vi "Read I16 analogue Data.vi"(6 "Block Header":string, 7 "Channel info":T1[](array[typedef]), 8 "Time Trace In":T2[](array[typedef]), 9 "Analogue Index":i32[](array[numeric]), 10 "pos offset (bytes:0)":i32, 11 "refnum":refnum<file>) -> (0 "Time Trace out":T2[](array[typedef]), 1 "EOF?":bool, 2 "mark after read (bytes)":i32)   [LabVIEW 2021]
uses:
  Controls/Time_Trace_Cluster.ctl
  Controls/Read I16 data cluster.ctl
  Globals/Meas_global.vi
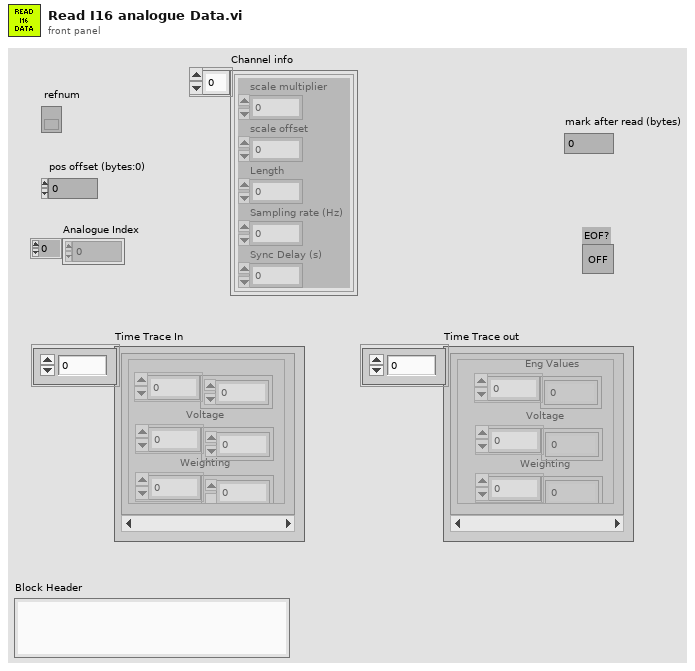
[diagram p1: front panel]
types:
  T1 = typedef "Read I16 data cluster.ctl" = cluster{"scale multiplier":dbl, "scale offset":dbl, "Length":i32, "Sampling rate (Hz)":dbl, "Sync Delay (s)":dbl}
  T2 = typedef "Time_Trace_Cluster.ctl" = cluster{"Weighting":dbl[], "Voltage":dbl[], "Eng Values":dbl[]}
  T3 = typedef "Analysis_info_cluster.ctl" = cluster{"Colour":u32, "Inst type":T4, "Inst name":string, "Symbol":string, "Code name":string, "Extra Info":string, "Inst Array":T5, "Extra Titles":string[], "Extra Values":string[], "U":dbl, "u^2":dbl, "u^3":dbl, "u^4":dbl, "Skew_u":dbl, "Kurt_u":dbl, "Sd Error in Mean":dbl, "% u'/U":dbl, "X":dbl, "Y":dbl, "Z":dbl, "Timescale integral Estimate":dbl, "Sd Error in Variance":dbl, "Calib File":path, "Calib Constants":dbl[], "Output Position":bool, "Stats":enum16{"None", "Basic", "Full"}, "Av Sampling Rate":dbl, "Av No of Samples":dbl, "Total Meas Time (s)":dbl, "ADAM Ch Name":string, "Max value":dbl, "Min value":dbl, "Req Sample Rate Hz":dbl, "Sync Delay Time (s)":dbl, "Ch No":i16, "Device":string, "Use Latest Calib":bool, "Port":string, "Metadata Ch Names":string[], "Metadata Ch Values":string[], "Label":string}
  T4 = typedef "Inst_type.ctl" = enum16{"Raw voltage", "Raw with zero offsetting", "Propeller anemometer", "Pressure Transducer", "Pitot-static tube", "Hot wire", "Cross wire 1", "Cross wire 2", "Generic Linear", "Generic Polynomial", "Generic BackPoly", "Fast FID", "Thermocouple", "Cold wire", "Pulsed Wire", "LDA Vel", "LDA Tran time", "LDA Arr time", "Microphone"}
  T5 = typedef "Instrument_Array.ctl" = enum16{"PWA", "LDA", "Analogue"}
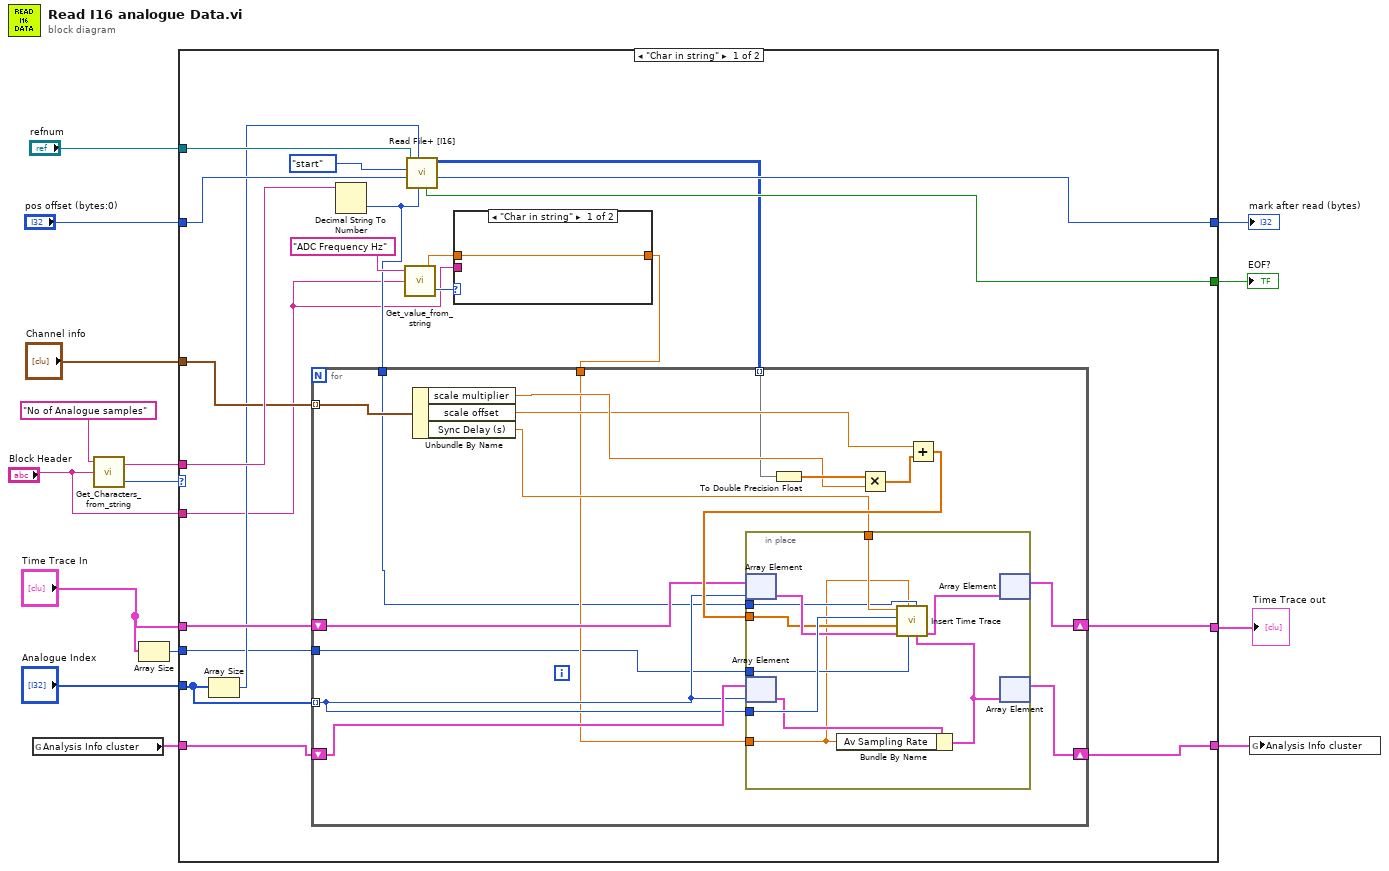
[diagram p0: block diagram]
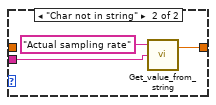
[diagram p2: hidden frame]
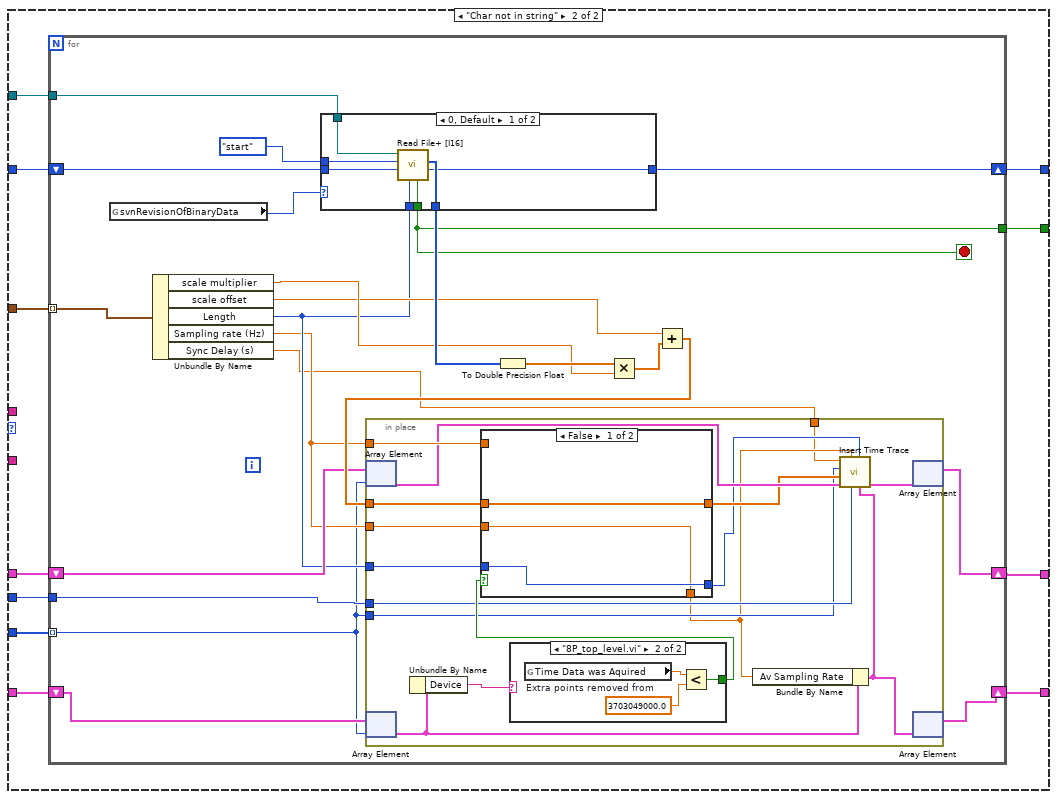
[diagram p3: hidden frame]
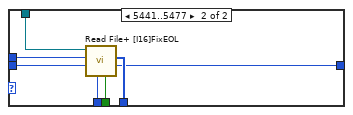
[diagram p4: hidden frame]
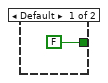
[diagram p5: hidden frame]
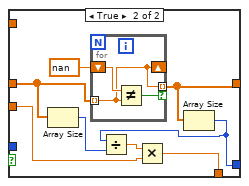
[diagram p6: hidden frame]
diagram:
  n1 = global read "Meas_global.vi" "Analysis Info cluster"() -> (w2:T3[])
  n2 = call "Get_Characters_from_string.vi"("Input string"="Block Header", "Variable name"="No of Analogue samples") -> ("Status"=w8:enum16{"Char in string", "Char not in string"}, "Value"=w7:string)  [unwired: 1 in]
  n3 = Array Size(array="Time Trace In") -> (size(s)=w3:i32)
  n4 = case shown="\"Char in string\"" w8 {
    tunnel: "Time Trace In" -> [w27 w77]
    tunnel: "Analogue Index" -> [w25 w70]
    tunnel: "Channel info" -> [w23 w76]
    tunnel: [w26 w75] -> w13
    tunnel: "pos offset (bytes:0)" -> [w32 w74]
    tunnel: [w31 w73] -> w11
    tunnel: "refnum" -> [w30 w72]
    tunnel: w7 -> [w29 _]
    tunnel: [w28 w71] -> w6
    tunnel: "Block Header" -> [w20 _]
    tunnel: w3 -> [w18 w69]
    tunnel: w2 -> [w17 w68]
    tunnel: [w16 w67] -> w1
    frame "Char in string" {
      n5 = Array Size(array=w25) -> (size(s)=w22:i32)
      n6 = Decimal String To Number(string=w29) -> (number=w21:i32)  [unwired: 3 out]
      n7 = call "Get_value_from_string.vi"("Input string"=w20, "Variable name"="ADC Frequency Hz") -> ("Status"=w35:enum16{"Char in string", "Char not in string"}, "Value"=w36:dbl)  [unwired: 1 in]
      n8 = call <vilib>:"Read File+ [I16].vi"("2D number of columns/1D count"=w21, "2D number of rows"=w22, "pos offset (bytes:0)"=w32, "pos mode (rel. to current:2)"=enum16{"start", "end", "current"}."start", "refnum"=w30) -> ("mark after read (bytes)"=w31:i32, "2D data"=w24:i16[][], "EOF?"=w28:bool)  [unwired: 1 in, 3 out]
      n9 = case shown="\"Char in string\"" w35 {
        tunnel: w36 -> [w63 _]
        tunnel: [w63 w64] -> w19
        tunnel: w20 -> [_ w65]
        frame "Char in string" {
        }
        frame "Char not in string" {
          n10 = call "Get_value_from_string.vi"("Input string"=w65, "Variable name"="Actual sampling rate") -> ("Value"=w64:dbl)  [unwired: 1 in, 1 out]
        }
      }
      n11 = for {
        shift-right: [w47] -> w26
        shift-left: w27 -> [w42]
        tunnel: w25 -> [w41] mode=indexing
        tunnel: w24 -> [w46] mode=indexing
        tunnel: w23 -> [w45] mode=indexing
        tunnel: w21 -> [w37]
        tunnel: w19 -> [w39]
        tunnel: w18 -> [w38]
        shift-right: [w43] -> w16
        shift-left: w17 -> [w44]
        n12 = Unbundle By Name(w45) -> ("scale multiplier"=w50:dbl, "scale offset"=w49:dbl, "Sync Delay (s)"=w40:dbl)
        n13 = To Double Precision Float(number=w46) -> (double precision float=w51:dbl[])
        n14 = Multiply(x=w51, y=w50) -> (x*y=w52:dbl[])
        n15 = Add(x=w49, y=w52) -> (x+y=w48:dbl[])
        n16 = in-place {
          in-place-border: w48 -> [w54]
          in-place-border: w39 -> [w53]
          in-place-border: w41 -> [w62]
          in-place-border: w40 -> [w61]
          in-place-border: w38 -> [w56]
          in-place-border: w37 -> [w55]
          n17 = in-place-array #1(w42, w41) -> (w60:T2)
          n18 = in-place-array #2(w44, w41) -> (w58:T3)
          n19 = Bundle By Name(cluster=w58, "Av Sampling Rate"=w53) -> (w57:T3)
          n20 = call "Insert Time Trace.vi"("Anlaysis Info Cluster"=w57, "No of Samples"=w55, "Total No of Chs"=w56, "Sampling Rate (Hz)"=w53, "Time Trace In"=w60, "Input Array"=w54, "Index"=w62, "Sync Delay (s)"=w61) -> ("Time Trace Out"=w59:T2)  [unwired: 3 in]
          n21 = in-place-array #1(w59) -> (w47:T2[])  [unwired: 1 out]
          n22 = in-place-array #2(w57) -> (w43:T3[])  [unwired: 1 out]
        }
      }
    }
    frame "Char not in string" {
      n23 = for {
        shift-right: [w91] -> w75
        shift-left: w77 -> [w92]
        tunnel: w70 -> [w79] mode=indexing
        tunnel: w76 -> [w90] mode=indexing
        shift-right: [w88] -> w73
        shift-left: w74 -> [w89]
        tunnel: w72 -> [w87]
        tunnel: [w86] -> w71
        tunnel: w69 -> [w81]
        shift-right: [w83] -> w67
        shift-left: w68 -> [w84]
        stop <- w86 stop-if-true
        n24 = global read "Meas_global.vi" "svnRevisionOfBinaryData"() -> (w82:u32)
        n25 = Unbundle By Name(w90) -> ("scale multiplier"=w95:dbl, "scale offset"=w94:dbl, "Length"=w85:i32, "Sampling rate (Hz)"=w80:dbl, "Sync Delay (s)"=w78:dbl)
        n26 = case shown="0, Default" w82 {
          tunnel: enum16{"start", "end", "current"}."start" ("pos mode (rel. to current:2)") -> [w106 w113]
          tunnel: [w105 w112] -> w96
          tunnel: w89 -> [w104 w111]
          tunnel: [w103 w110] -> w88
          tunnel: w87 -> [w102 w109]
          tunnel: [w101 w108] -> w86
          tunnel: w85 -> [w100 w107]
          frame 0, Default {
            n27 = call <vilib>:"Read File+ [I16].vi"("2D number of columns/1D count"=w100, "pos offset (bytes:0)"=w104, "pos mode (rel. to current:2)"=w106, "refnum"=w102) -> ("mark after read (bytes)"=w103:i32, "1D data"=w105:i16[], "EOF?"=w101:bool)  [unwired: 2 in, 3 out]
          }
          frame 5441..5477 {
            n28 = call "Read File+ [I16]FixEOL.vi"("2D number of columns/1D count"=w107, "pos offset (bytes:0)"=w111, "pos mode (rel. to current:2)"=w113, "refnum"=w109) -> ("mark after read (bytes)"=w110:i32, "1D data"=w112:i16[], "EOF?"=w108:bool)  [unwired: 3 in, 2 out]
          }
        }
        n29 = To Double Precision Float(number=w96) -> (double precision float=w97:dbl[])
        n30 = Multiply(x=w97, y=w95) -> (x*y=w98:dbl[])
        n31 = Add(x=w94, y=w98) -> (x+y=w93:dbl[])
        n32 = in-place {
          in-place-border: w93 -> [w127]
          in-place-border: w85 -> [w128]
          in-place-border: w80 -> [w126]
          in-place-border: w81 -> [w119]
          in-place-border: w80 -> [w125]
          in-place-border: w79 -> [w117]
          in-place-border: w78 -> [w114]
          n33 = in-place-array #3(w92, w79) -> (w122:T2)
          n34 = in-place-array #4(w84, w79) -> (w129:T3)
          n35 = Unbundle By Name(w129) -> ("Device"=w124:string)
          n36 = case shown="\"8P_top_level.vi\"" w124 {
            tunnel: [FALSE w131] -> w123
            frame Default {
            }
            frame "8P_top_level.vi" {
              w132 = 3703049000.0  # Extra points removed from
              n37 = global read "Meas_global.vi" "Time Data was Aquired"() -> (w133:dbl)
              n38 = Less?(x=w133, y=w132) -> (x < y?=w131:bool)
            }
          }
          n39 = case shown="False" w123 {
            tunnel: w128 -> [w135 _]
            tunnel: [w135 w137] -> w115
            tunnel: w127 -> [w136 w142]
            tunnel: [w136 w143] -> w118
            tunnel: [w134 w138] -> w116
            tunnel: w126 -> [w134 w139]
            tunnel: w125 -> [_ _]
            frame False {
            }
            frame True {
              n40 = Array Size(array=w142) -> (size(s)=w141:i32)
              n41 = for {
                shift-right: [w146] -> _
                shift-left: nan -> [w147]
                tunnel: w142 -> [w146] mode=indexing
                tunnel: [w146] -> w143 mode=indexing if=w145
                n42 = Not Equal?(x=w147, y=w146) -> (x != y?=w145:bool)
              }
              n43 = Array Size(array=w143) -> (size(s)=w137:i32)
              n44 = Divide(x=w137, y=w141) -> (x/y=w140:dbl)
              n45 = Multiply(x=w140, y=w139) -> (x*y=w138:dbl)
            }
          }
          n46 = Bundle By Name(cluster=w129, "Av Sampling Rate"=w116) -> (w120:T3)
          n47 = call "Insert Time Trace.vi"("Anlaysis Info Cluster"=w120, "No of Samples"=w115, "Total No of Chs"=w119, "Sampling Rate (Hz)"=w116, "Time Trace In"=w122, "Input Array"=w118, "Index"=w117, "Sync Delay (s)"=w114) -> ("Time Trace Out"=w121:T2)  [unwired: 3 in]
          n48 = in-place-array #3(w121) -> (w91:T2[])  [unwired: 1 out]
          n49 = in-place-array #4(w120) -> (w83:T3[])  [unwired: 1 out]
        }
      }
    }
  }
  "Time Trace out" <- w13
  "mark after read (bytes)" <- w11
  "EOF?" <- w6
  n50 = global write "Meas_global.vi" "Analysis Info cluster"(w1) -> ()
